vi "Create Orchestration.vi"(6 "timeout (ms)":i32=5000, 8 "error in":errorcluster, 10 "Orchestration Config":T1, 11 "gRPC ID in":T3) -> (0 "error out":errorcluster, 2 "Orchestration Script":string, 3 "gRPC ID out":T3)   [LabVIEW 2021, in "CIFManagerClientWrapper.lvlib"]
uses:
  CIFManagerClientWrapper.lvlib
  <vilib>/gRPC/LabVIEW gRPC Library/Shared/grpcId.ctl
  CIF_Manager_client/RPC Messages/cif_manager_CreateOrchRequest.ctl
  CIF_Manager_client/RPC Messages/cif_manager_OrchestrationLanguage.ctl
  CIF_Manager_client/CIF_Manager_client.lvlib
  <vilib>/gRPC/LabVIEW gRPC Library/grpc-lvsupport-release.lvlib
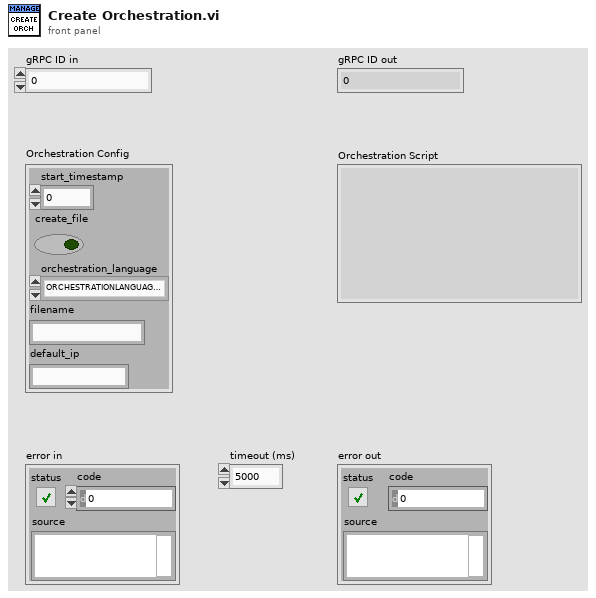
[diagram p1: front panel]
types:
  T1 = typedef "CIF_Manager_client.lvlib/cif_manager_CreateOrchRequest.ctl" = cluster{"start_timestamp":u64, "create_file":bool, "orchestration_language":T2, "filename":string, "default_ip":string}
  T2 = typedef "CIF_Manager_client.lvlib/cif_manager_OrchestrationLanguage.ctl" = enum32{"ORCHESTRATIONLANGUAGE_UNKNOWN", "ORCHESTRATIONLANGUAGE_PYTHON"}
  T3 = typedef "grpc-lvsupport-release.lvlib/grpcId.ctl" = u64
  T4 = typedef "CIF_Manager_client.lvlib/cif_manager_CreateOrchResponse.ctl" = cluster{"orchestration_script":string, "status":T5}
  T5 = typedef "CIF_Manager_client.lvlib/cif_common_Status.ctl" = cluster{"code":i32, "message":string}
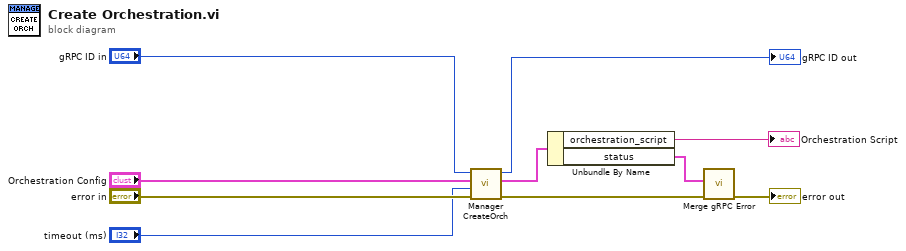
[diagram p0: block diagram]
diagram:
  n1 = call "Manager CreateOrch.vi"("error in"="error in", "timeout (ms)"="timeout (ms)", "Request Data"="Orchestration Config", "gRPC ID"="gRPC ID in") -> ("error out"=w6:errorcluster, "Response Data"=w4:T4, "gRPC ID out"=→"gRPC ID out":T3)  [unwired: 5 in]
  n2 = Unbundle By Name(w4) -> ("orchestration_script"=→"Orchestration Script":string, "status"=w3:T5)
  n3 = call "Merge gRPC Error.vi"("error in (no error)"=w6, "gRPC Error"=w3) -> ("error out"=→"error out":errorcluster)  [unwired: 9 in]
